vi "Write Refresh Time.vi"(8 "error in (no error)":errorcluster, 10 "Refresh Time (ms)":i32, 11 "Transport in":refnum<class "Transport.lvclass">) -> (0 "error out":errorcluster, 3 "Transport out":refnum<class "Transport.lvclass">)   [LabVIEW 2019, in "Transport.lvclass"]
uses:
  Transport.lvclass
  Transport.lvclass/Transport.ctl
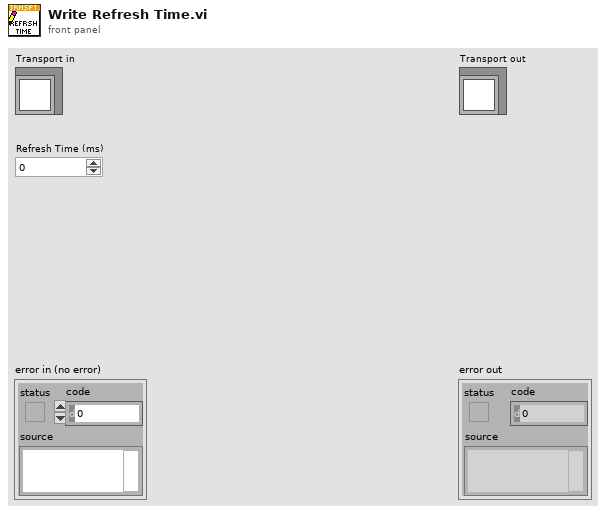
[diagram p1: front panel]
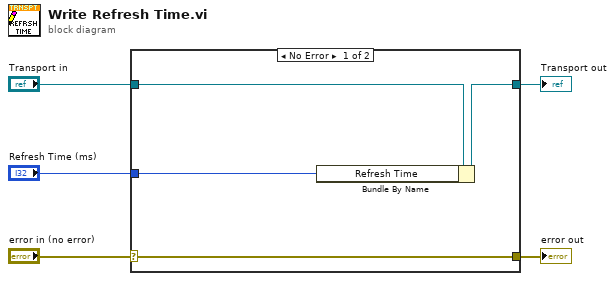
[diagram p0: block diagram]
diagram:
  n1 = case shown="No Error" "error in (no error)" {
    selector: "error in (no error)" -> [w9 w10]
    tunnel: [w9 w10] -> w4
    tunnel: [w7 w11] -> w2
    tunnel: "Transport in" -> [w8 w11]
    tunnel: "Refresh Time (ms)" -> [w6 _]
    frame No Error {
      n2 = Bundle By Name(cluster=w8, "Refresh Time"=w6) -> (w7:refnum<class "Transport.lvclass">)
    }
    frame Error {
    }
  }
  "error out" <- w4
  "Transport out" <- w2
